vi "add model to project.vi"(8 "error in":errorcluster, 10 "VI path":path, 11 "completed project":path) -> (0 "error out":errorcluster)   [LabVIEW 2014, in "CD model script.lvlib"]
uses:
  CD model script.lvlib
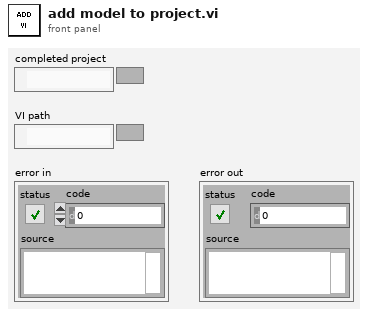
[diagram p1: front panel]
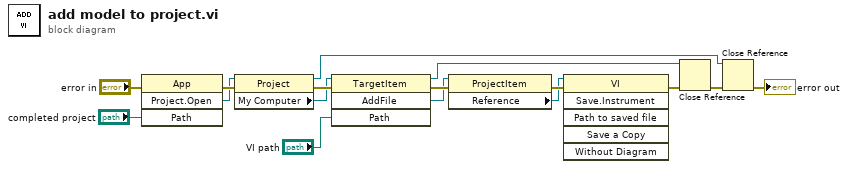
[diagram p0: block diagram]
diagram:
  n1 = invoke class="App" method="Project.Open"(error in="error in", "Path"="completed project") -> (error out=w15:errorcluster, "Project:Open"=w11:refnum<vi>)  [unwired: 2 in, 2 out]
  n2 = property class="Project"(reference=w11, error in=w15) -> (reference out=w5:refnum<vi>, error out=w12:errorcluster, "My Computer"=w10:refnum<vi>)
  n3 = invoke class="TargetItem" method="AddFile"(reference=w10, error in=w12, "Path"="VI path") -> (reference out=w7:refnum<vi>, error out=w13:errorcluster, "AddFile"=w2:refnum<vi>)  [unwired: 1 in, 1 out]
  n4 = property class="ProjectItem"(reference=w2, error in=w13) -> (error out=w3:errorcluster, "Reference"=w1:refnum<vi>)  [unwired: 1 out]
  n5 = invoke class="VI" method="Save.Instrument"(reference=w1, error in=w3) -> (error out=w4:errorcluster)  [unwired: 4 in, 5 out]
  n6 = Close Reference(reference=w7, error in (no error)=w4) -> (error out=w8:errorcluster)
  n7 = Close Reference(reference=w5, error in (no error)=w8) -> (error out=→"error out":errorcluster)
